vi "Запись волны.vi"() -> ()   [LabVIEW 2017]
panel:
  out "Waveform Chart":cluster{dbl, dbl}(graph)
  in  "stop":bool
  in  "file path (use dialog)":path
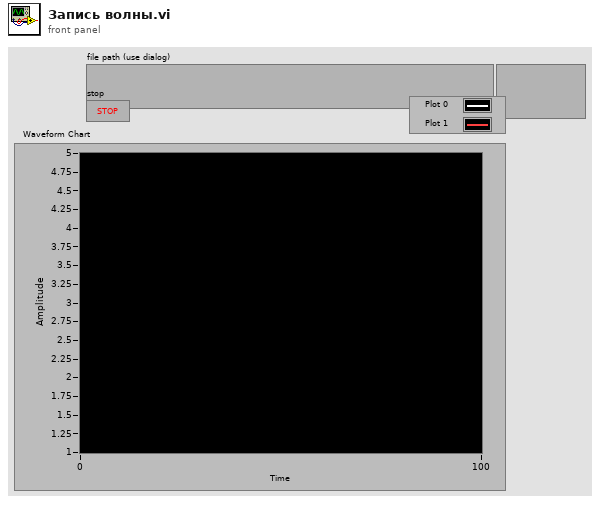
[diagram p1: front panel]
types:
  T1 = enum16{"open", "replace", "create", "open or create", "replace or create", "replace or create with confirmation"}
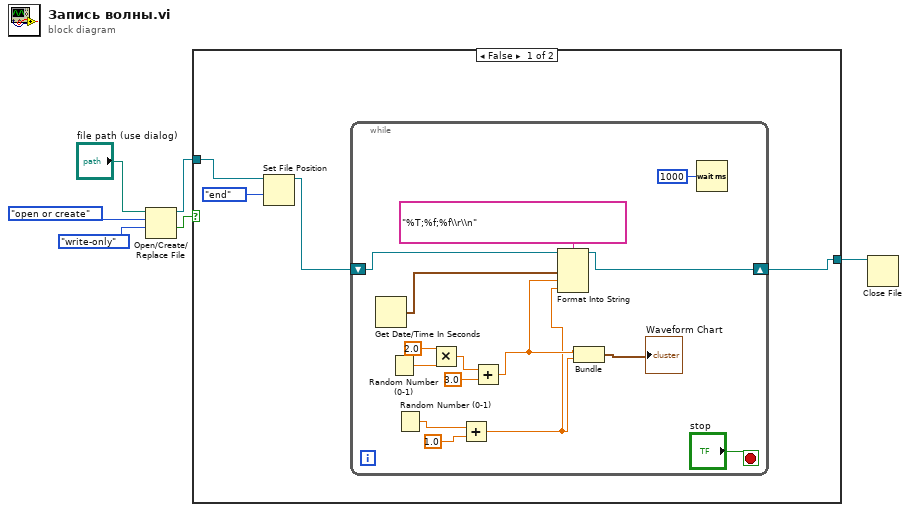
[diagram p0: block diagram]
diagram:
  n1 = Open/Create/Replace File(file path (use dialog)="file path (use dialog)", operation (0:open)=T1."open or create", access (0:read/write)=enum16{"read/write", "read-only", "write-only"}."write-only") -> (refnum out=w2:refnum<file>, cancelled=w3:bool)  [unwired: 3 in, 1 out]
  n2 = case shown="False" w3 {
    tunnel: w2 -> [w10 w26]
    tunnel: [w7 w26] -> w1
    frame False {
      n3 = Set File Position(refnum=w10, from (0:start)=enum16{"start", "end", "current"}."end") -> (refnum out=w8:refnum<file>)  [unwired: 2 in, 1 out]
      n4 = while {
        shift-right: [w14] -> w7
        shift-left: w8 -> [w24]
        stop <- "stop" stop-if-true
        n5 = Get Date/Time In Seconds() -> (seconds since 1Jan1904=w21:timestamp)
        n6 = Random Number (0-1)() -> (number: 0 to 1=w18:dbl)
        n7 = Random Number (0-1)() -> (number: 0 to 1=w20:dbl)
        n8 = Multiply(x=2.0, y=w18) -> (x*y=w16:dbl)
        n9 = Add(x=w20, y=1.0) -> (x+y=w11:dbl)
        n10 = Add(x=w16, y=3.0) -> (x+y=w12:dbl)
        n11 = Format Into String(format string="%T;%f;%f\\r\\n", initial string=w24, w21, w12, w11) -> (resulting string=w14:refnum<file>)  [unwired: 1 in, 1 out]
        n12 = Bundle(w12, w11) -> (→"Waveform Chart":cluster{dbl, dbl})  [unwired: 1 in]
        n13 = Wait (ms)(milliseconds to wait=u32 1000) -> ()  [unwired: 1 out]
      }
    }
    frame True {
    }
  }
  n14 = Close File(refnum=w1) -> ()  [unwired: 1 in, 2 out]
